vi "Get AI Ref.vi"(8 "Error In":errorcluster, 11 "LINX Device Config":T1) -> (0 "Error Out":errorcluster, 2 "AI Ref":dbl, 3 "LINX Device Config":T1)   [LabVIEW 2011, in "LVH-LINX.lvlib" / "Device.lvlib"]
uses:
  Device.lvlib
  Type Defs/LINX Device Config.ctl
  Type Defs/Interface.ctl
  Type Defs/TCP Config.ctl
  Type Defs/Channels.ctl
  Type Defs/Error Type.ctl
  LVH-LINX.lvlib
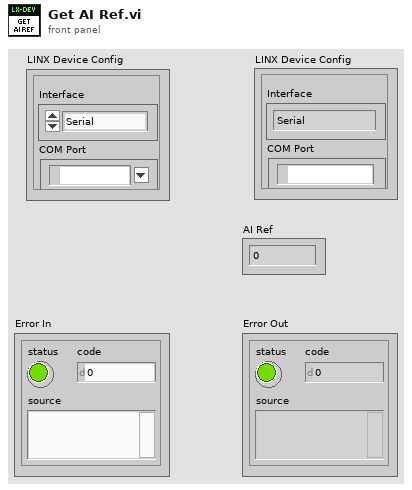
[diagram p1: front panel]
types:
  T1 = typedef "LVH-LINX.lvlib/Device.lvlib/LINX Device Config.ctl" = cluster{"Interface":T2, "COM Port":refnum<visa-resource-name>, "TCP Configuration":T3, "Device Family":u8, "Device ID":u8, "Device Name":string, "TCP Ref":refnum<k5>, "Channels":T4}
  T2 = typedef "LVH-LINX.lvlib/Interface.ctl" = enum16{"Serial", "TCP"}
  T3 = typedef "LVH-LINX.lvlib/Device.lvlib/TCP Config.ctl" = cluster{"IP Address":string, "Port":u16}
  T4 = typedef "LVH-LINX.lvlib/Channels.ctl" = cluster{"DI":u8[], "DO":u8[], "AI":u8[], "AO":u8[], "PWM":u8[], "QE":u8[], "UART":u8[], "I2C 2":u8[], "SPI":u8[], "CAN":u8[], "Servo":u8[], "AI Ref (V)":dbl, "AO Ref (V)":dbl, "AO Resolution (Bits)":u8}
  T5 = typedef "LVH-LINX.lvlib/Error Type.ctl" = enum16{"Unknown", "Timeout", "Corrupt Return Packet", "Unable To Connect", "Command Not Supported", "Channel DNE", "Invalid COM Config", "Firmware Version Mismatch", "myRIO Support", "CMD Specific Error"}
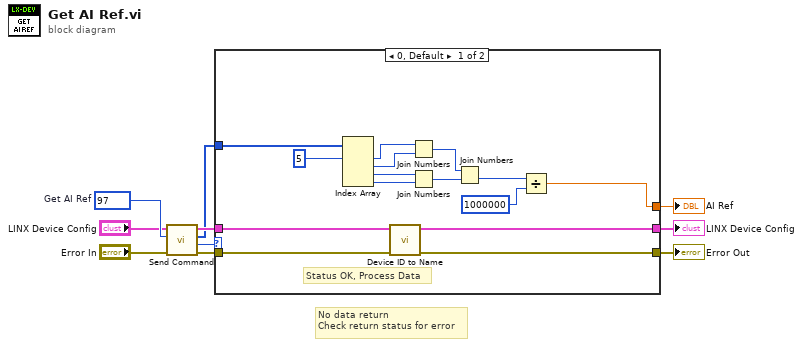
[diagram p0: block diagram]
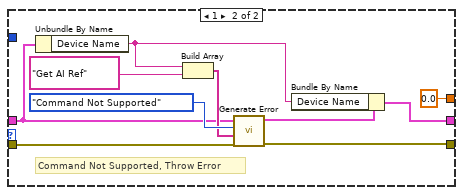
[diagram p2: hidden frame]
diagram:
  w9 = u16 97  # Get AI Ref
  # "No data return\nCheck return status for error"
  n1 = call "Send Command.vi"("Error In"="Error In", "CMD"=w9, "LINX Device Config"="LINX Device Config") -> ("Error Out"=w4:errorcluster, "Status"=w2:u8, "Response"=w3:u8[], "LINX Device Config"=w6:T1)  [unwired: 5 in]
  n2 = case shown="0, Default" w2 {
    tunnel: [w22 w29] -> w7
    tunnel: w6 -> [w25 w28]
    tunnel: [w23 w34] -> w5
    tunnel: w4 -> [w24 w35]
    tunnel: w3 -> [w21 _]
    tunnel: [w11 0.0] -> w1
    frame 0, Default {
      # "Status OK, Process Data"
      n3 = Index Array(array=w21, index #1=5 ("index")) -> (element #1=w19:u8, element #2=w18:u8, element #3=w16:u8, element #4=w15:u8)  [unwired: 3 in]
      n4 = call "Device ID to Name.vi"("Error In"=w24, "LINX Device Config"=w25) -> ("Error Out"=w23:errorcluster, "LINX Device Config"=w22:T1)  [unwired: 7 in, 1 out]
      n5 = Join Numbers(hi=w19, lo=w18) -> ((hi.lo)=w17:u16)
      n6 = Join Numbers(hi=w16, lo=w15) -> ((hi.lo)=w14:u16)
      n7 = Join Numbers(hi=w17, lo=w14) -> ((hi.lo)=w13:u32)
      n8 = Divide(x=w13, y=u32 1000000) -> (x/y=w11:dbl)
    }
    frame 1 {
      # "Command Not Supported, Throw Error"
      n9 = Unbundle By Name(w28) -> ("Device Name"=w27:string)
      n10 = Build Array(w27, "Get AI Ref") -> (w31:string[])
      n11 = call "Generate Error.vi"("Error In"=w35, "Arguments"=w31, "Error Type"=Error_Type."Command Not Supported", "LINX Device Config"=w28) -> ("Error Out"=w34:errorcluster, "LINX Device Config"=w30:T1)  [unwired: 6 in]
      n12 = Bundle By Name(cluster=w30, "Device Name"=w27) -> (w29:T1)
    }
  }
  "Error Out" <- w5
  "LINX Device Config" <- w7
  "AI Ref" <- w1
